vi "sv_Enumeration (Direction).vi"() -> (2 "direction strings":string[](array[string]), 3 "direction values":T1[](array[typedef])=[-6, -5, -4, -3, -2, -1, 0, 1, 2, 3, 4, 5, 6] items=["-Z Rotation"=-6, "-Y Rotation"=-5, "-X Rotation"=-4, "-Z Translation"=-3, "-Y Translation"=-2, "-X Translation"=-1, "Scalar"=0, "+X Translation"=1, "+Y Translation"=2, "+Z Translation"=3, "+X Rotation"=4, "+Y Rotation"=5, "+Z Rotation"=6])   [LabVIEW 2017, in "SoundVib_UFF58.lvlib"]
uses:
  <vilib>/addons/Sound and Vibration/svt_UFF58/SoundVib_UFF58.lvlib
  <vilib>/addons/Sound and Vibration/svt_UFF58/subVIs/sv_UFF58 Response Direction.ctl
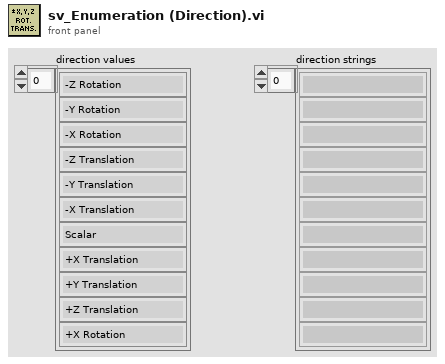
[diagram p1: front panel]
types:
  T1 = typedef "SoundVib_UFF58.lvlib/sv_UFF58 Response Direction.ctl" = i32
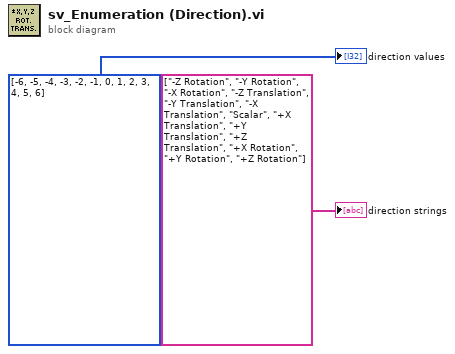
[diagram p0: block diagram]
diagram:
  w1 = T1[] [-6, -5, -4, -3, -2, -1, 0, 1, 2, 3, 4, 5, 6] items=["-Z Rotation"=-6, "-Y Rotation"=-5, "-X Rotation"=-4, "-Z Translation"=-3, "-Y Translation"=-2, "-X Translation"=-1, "Scalar"=0, "+X Translation"=1, "+Y Translation"=2, "+Z Translation"=3, "+X Rotation"=4, "+Y Rotation"=5, "+Z Rotation"=6]
  "direction strings" <- string[] ["-Z Rotation", "-Y Rotation", "-X Rotation", "-Z Translation", "-Y Translation", "-X Translation", "Scalar", "+X Translation", "+Y Translation", "+Z Translation", "+X Rotation", "+Y Rotation", "+Z Rotation"] ("ResponseDirection")
  "direction values" <- w1
